vi "GV_PlotLscale.vi"(8 "error in (no error)":errorcluster, 11 "Gviewer in":refnum<class "Gviewer.lvclass">) -> (0 "error out":errorcluster, 3 "Gviewer out":refnum<class "Gviewer.lvclass">)   [LabVIEW 2020, in "Sgraph_lib_V1.lvlib" / "Gviewer.lvclass"]
doc: "Andre Koelewijn, 10 feb 2022,\n\nPlot Left Lscale data if used"
uses:
  Gviewer.lvclass
  Gviewer.lvclass/Gviewer.ctl
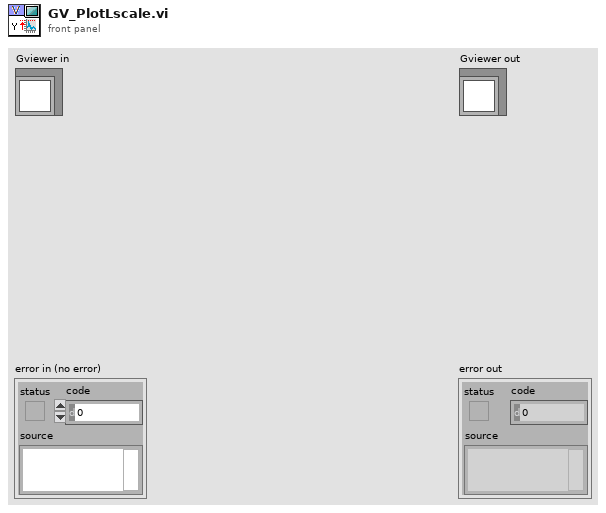
[diagram p1: front panel]
types:
  T1 = typedef "Sgraph_lib_V1.lvlib/Gviewer.lvclass/TD_Lscale.ctl" = enum16{"none", "one", "many"}
  T2 = typedef "Sgraph_lib_V1.lvlib/Gviewer.lvclass/AutoScale.ctl" = enum16{"FitEqual", "FitMax", "StackEqual", "StackMax", "StackPerType"}
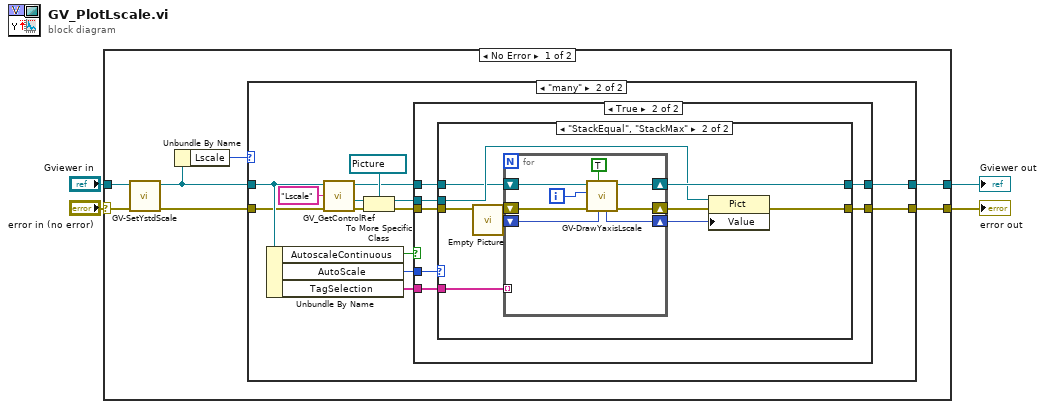
[diagram p0: block diagram]
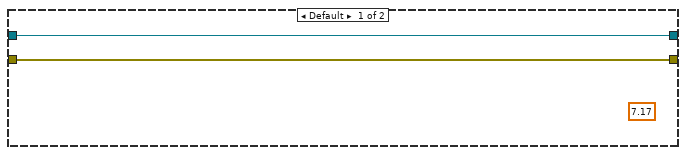
[diagram p2: hidden frame]
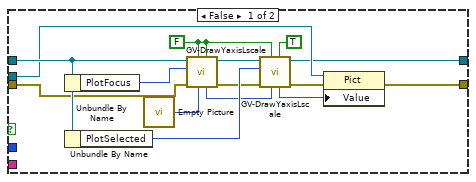
[diagram p3: hidden frame]
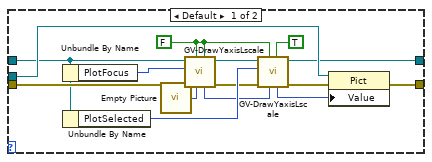
[diagram p4: hidden frame]
diagram:
  n1 = case shown="No Error" "error in (no error)" {
    selector: "error in (no error)" -> [w6 w83]
    tunnel: [w9 w83] -> w3
    tunnel: [w10 w82] -> w1
    tunnel: "Gviewer in" -> [w7 w82]
    frame No Error {
      n2 = call "GV-SetYstdScale.vi"("error in (no error)"=w6, "Gviewer in"=w7) -> ("error out"=w5:errorcluster, "Gviewer out"=w8:refnum<class "Gviewer.lvclass">)  [unwired: 8 in]
      n3 = Unbundle By Name(w8) -> ("Lscale"=w11:T1)
      n4 = case shown="\"many\"" w11 {
        tunnel: w8 -> [w13 w17]
        tunnel: [w13 w26] -> w10
        tunnel: [w12 w24] -> w9
        tunnel: w5 -> [w12 w14]
        frame Default {
          (unwired) 7.17 ("num")
        }
        frame "many" {
          n5 = Unbundle By Name(w17) -> ("AutoscaleContinuous"=w23:bool, "AutoScale"=w25:T2, "TagSelection"=w27:string[])
          n6 = call "GV_GetControlRef.vi"("error in (no error)"=w14, "CNT name"="Lscale", "Gviewer in"=w17) -> ("error out"=w22:errorcluster, "Reference"=w21:refnum<vi>, "Gviewer out"=w18:refnum<class "Gviewer.lvclass">)  [unwired: 6 in]
          n7 = To More Specific Class(target class=refnum<vi> refnum ("2D Picture"), reference=w21, error in=w22) -> (specific class reference=w15:refnum<vi>, error out=w16:errorcluster)
          n8 = case shown="True" w23 {
            tunnel: w27 -> [_ w49]
            tunnel: w18 -> [w32 w48]
            tunnel: [w29 w47] -> w26
            tunnel: w25 -> [_ w46]
            tunnel: [w28 w45] -> w24
            tunnel: w16 -> [w31 w44]
            tunnel: w15 -> [w30 w43]
            frame False {
              w33 = FALSE ("Stacked?")
              n9 = Unbundle By Name(w32) -> ("PlotFocus"=w42:i32)
              n10 = Unbundle By Name(w32) -> ("PlotSelected"=w40:i32)
              n11 = call "Empty Picture"() -> ("empty picture"=w35:picture)
              n12 = call "GV-DrawYaxisLscale.vi"("Dir"=w33, "Picture IN"=w35, "Stacked?"=w33, "error in (no error)"=w31, "Plot"=w42, "Gviewer in"=w32) -> ("error out"=w39:errorcluster, "Gviewer out"=w41:refnum<class "Gviewer.lvclass">, "Picture OUT"=w37:picture)  [unwired: 3 in]
              n13 = call "GV-DrawYaxisLscale.vi"("Dir"=TRUE ("Stacked?"), "Picture IN"=w37, "Stacked?"=w33, "error in (no error)"=w39, "Plot"=w40, "Gviewer in"=w41) -> ("error out"=w38:errorcluster, "Gviewer out"=w29:refnum<class "Gviewer.lvclass">, "Picture OUT"=w36:picture)  [unwired: 3 in]
              n14 = property class="Pict"(reference=w30, error in=w38, "Value"=w36) -> (error out=w28:errorcluster)  [unwired: 1 out]
            }
            frame True {
              n15 = case shown="\"StackEqual\", \"StackMax\"" w46 {
                tunnel: w49 -> [_ w66]
                tunnel: w48 -> [w60 w65]
                tunnel: [w58 w73] -> w47
                tunnel: [w61 w69] -> w45
                tunnel: w44 -> [w63 w67]
                tunnel: w43 -> [w62 w68]
                frame Default {
                  w51 = FALSE ("Stacked?")
                  n16 = Unbundle By Name(w60) -> ("PlotFocus"=w64:i32)
                  n17 = Unbundle By Name(w60) -> ("PlotSelected"=w57:i32)
                  n18 = call "Empty Picture"() -> ("empty picture"=w52:picture)
                  n19 = call "GV-DrawYaxisLscale.vi"("Dir"=w51, "Picture IN"=w52, "Stacked?"=w51, "error in (no error)"=w63, "Plot"=w64, "Gviewer in"=w60) -> ("error out"=w56:errorcluster, "Gviewer out"=w59:refnum<class "Gviewer.lvclass">, "Picture OUT"=w54:picture)  [unwired: 3 in]
                  n20 = call "GV-DrawYaxisLscale.vi"("Dir"=TRUE ("Stacked?"), "Picture IN"=w54, "Stacked?"=w51, "error in (no error)"=w56, "Plot"=w57, "Gviewer in"=w59) -> ("error out"=w55:errorcluster, "Gviewer out"=w58:refnum<class "Gviewer.lvclass">, "Picture OUT"=w53:picture)  [unwired: 3 in]
                  n21 = property class="Pict"(reference=w62, error in=w55, "Value"=w53) -> (error out=w61:errorcluster)  [unwired: 1 out]
                }
                frame "StackEqual", "StackMax" {
                  n22 = call "Empty Picture"() -> ("empty picture"=w72:picture)
                  n23 = for {
                    shift-right: [w80] -> w73
                    shift-left: w65 -> [w81]
                    shift-right: [w78] -> w71
                    shift-left: w72 -> [w79]
                    shift-right: [w75] -> w70
                    shift-left: w67 -> [w76]
                    tunnel: w66 -> [_] mode=indexing
                    i -> [w77]
                    n24 = call "GV-DrawYaxisLscale.vi"("Picture IN"=w79, "Stacked?"=TRUE, "error in (no error)"=w76, "Plot"=w77, "Gviewer in"=w81) -> ("error out"=w75:errorcluster, "Gviewer out"=w80:refnum<class "Gviewer.lvclass">, "Picture OUT"=w78:picture)  [unwired: 4 in]
                  }
                  n25 = property class="Pict"(reference=w68, error in=w70, "Value"=w71) -> (error out=w69:errorcluster)  [unwired: 1 out]
                }
              }
            }
          }
        }
      }
    }
    frame Error {
    }
  }
  "error out" <- w3
  "Gviewer out" <- w1
